vi "TDMS Read Channel Fields.vi"(4 "MN":string, 6 "SN":string, 7 "Group Name":string, 8 "error in (no error)":errorcluster, 9 "Channel":string, 10 "Custom Field Records to Search":string[](array[string]), 11 "tdms file ref":refnum<k34>) -> (0 "error out":errorcluster, 2 "Custom Fields":T1[](array[typedef]), 3 "tdms file ref":refnum<k34>)   [LabVIEW 2011]
uses:
  database/Fields/Field Record.ctl
  database/Fields/Field DataTypes.ctl
  database/Fields/Field NextItem.ctl
panel:
  out "x-y 2":u32
  out "x-y":u32
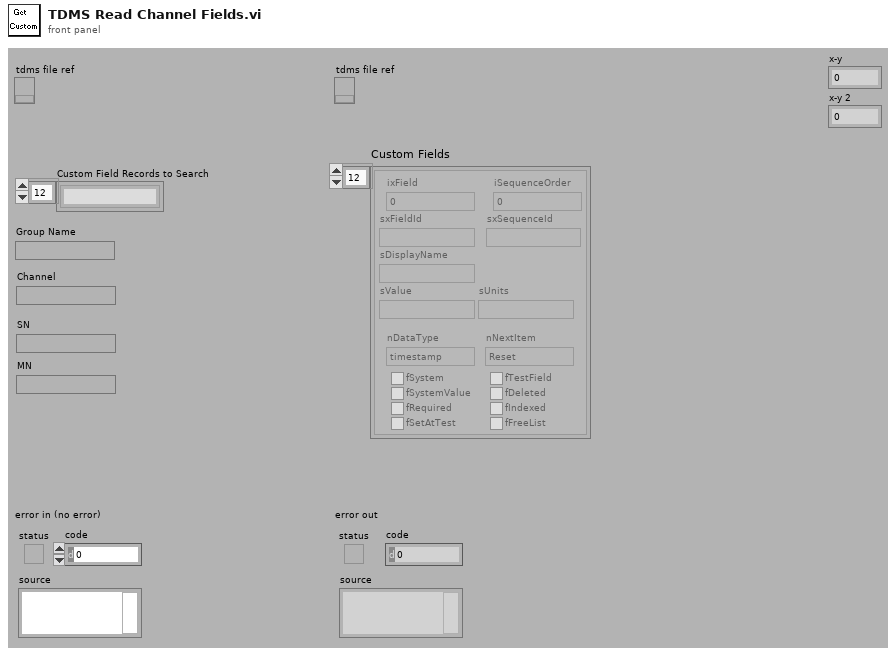
[diagram p1: front panel]
types:
  T1 = typedef "Field Record.ctl" = cluster{"ixField":i32, "iSequenceOrder":i32, "sxFieldId":string, "sxSequenceId":string, "sDisplayName":string, "sValue":string, "sUnits":string, "nDataType":T2, "nNextItem":T3, "fSystem":bool, "fSystemValue":bool, "fRequired":bool, "fSetAtTest":bool, "fTestField":bool, "fDeleted":bool, "fIndexed":bool, "fFreeList":bool}
  T2 = typedef "Field DataTypes.ctl" = enum32{"text", "numeric", "list", "timestamp", "boolean"}
  T3 = typedef "Field NextItem.ctl" = enum32{"Reset", "Retain", "Auto-Increment"}
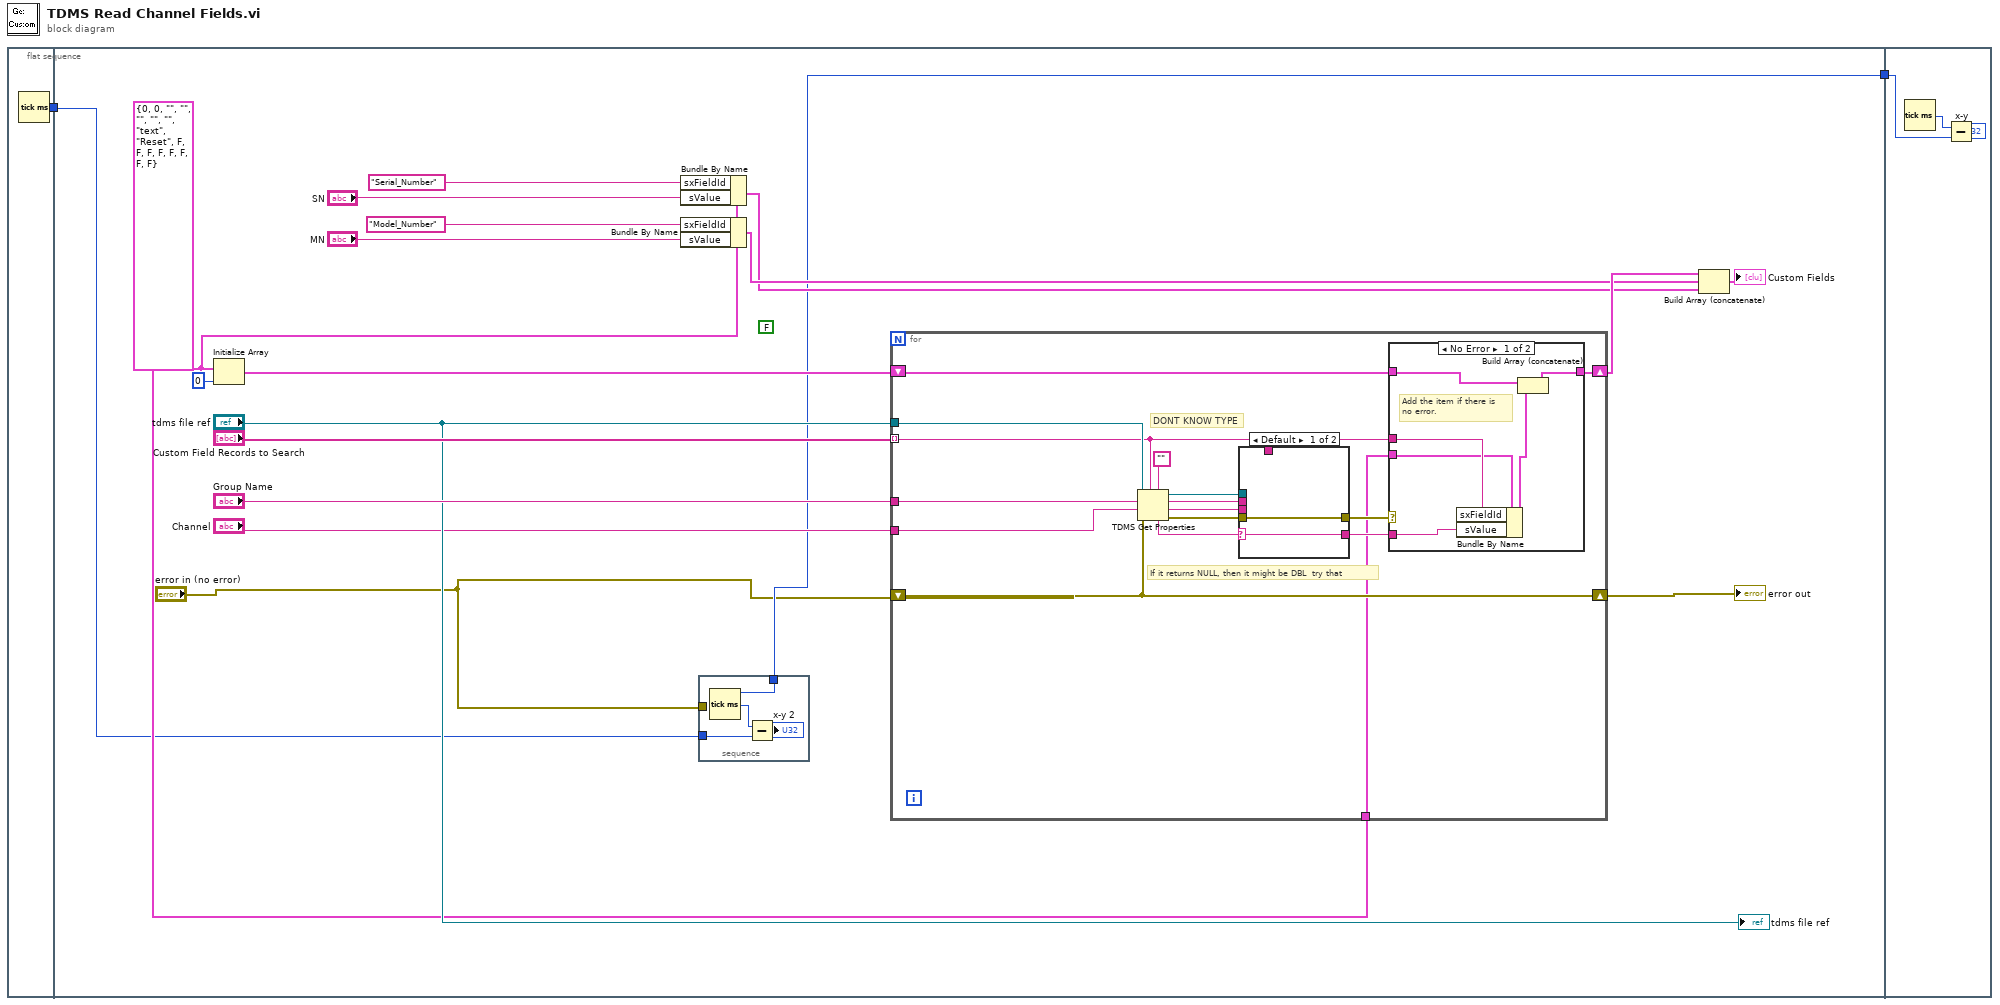
[diagram p0: block diagram]
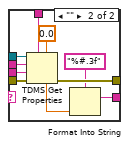
[diagram p2: hidden frame]
diagram:
  n1 = flat-sequence {
    tunnel: [w3] -> w1
    tunnel: [w6] -> w2
    tunnel: w1 -> [w5]
    tunnel: w2 -> [w62]
    frame #0 {
      n2 = Tick Count (ms)() -> (millisecond timer value=w3:u32)
    }
    frame #1 {
      (unwired) FALSE
      w15 = T1 {"ixField"=0, "iSequenceOrder"=0, "sxFieldId"="", "sxSequenceId"="", "sDisplayName"="", "sValue"="", "sUnits"="", "nDataType"=enum."text", "nNextItem"=enum."Reset", "fSystem"=FALSE, "fSystemValue"=FALSE, "fRequired"=FALSE, "fSetAtTest"=FALSE, "fTestField"=FALSE, "fDeleted"=FALSE, "fIndexed"=FALSE, "fFreeList"=FALSE} ("Field Record")
      n3 = Initialize Array(w15, 0 ("dimension size")) -> (w22:T1[])
      n4 = Bundle By Name(cluster=w15, "sxFieldId"="Serial_Number", "sValue"="SN") -> (w7:T1)
      n5 = Bundle By Name(cluster=w15, "sxFieldId"="Model_Number", "sValue"="MN") -> (w8:T1)
      n6 = stacked-sequence {
        tunnel: "error in (no error)" -> [_]
        tunnel: [w60] -> w6
        tunnel: w5 -> [w59]
        frame #0 {
          n7 = Tick Count (ms)() -> (millisecond timer value=w60:u32)
          n8 = Subtract(x=w60, y=w59) -> (x-y=→"x-y 2":u32)
        }
      }
      n9 = for {
        shift-right: [w36] -> w20
        shift-left: "error in (no error)" -> [w36]
        shift-right: [w37] -> w9
        shift-left: w22 -> [w38]
        tunnel: "tdms file ref" -> [w33]
        tunnel: "Custom Field Records to Search" -> [w30] mode=indexing
        tunnel: "Group Name" -> [w34]
        tunnel: w15 -> [w29]
        tunnel: "Channel" -> [w31]
        # "DONT KNOW TYPE"
        # "If it returns NULL, then it might be DBL  try that"
        n10 = TDMS Get Properties(5:"", 7:w30, 8:w36, 9:w31, 10:w34, 11:w33) -> (0:w27:errorcluster, 1:w23:string, 2:w24:string, 3:w26:refnum<k34>, 4:w25:string)  [unwired: 1 out]
        n11 = case shown="Default" w25 {
          selector: w25 -> [w39 _]
          tunnel: w27 -> [w40 w50]
          tunnel: w26 -> [_ w49]
          tunnel: w30 -> [_ w48]
          tunnel: [w40 w47] -> w32
          tunnel: [w39 w44] -> w35
          tunnel: w24 -> [_ w43]
          tunnel: w23 -> [_ w42]
          frame Default {
          }
          frame "" {
            n12 = TDMS Get Properties(5:0.0, 7:w48, 8:w50, 9:w42, 10:w43, 11:w49) -> (0:w47:errorcluster, 4:w46:dbl)  [unwired: 4 out]
            n13 = Format Into String(format string="%#.3f", w46) -> (resulting string=w44:string)  [unwired: 2 in, 1 out]
          }
        }
        n14 = case shown="No Error" w32 {
          tunnel: w38 -> [w56 w57]
          tunnel: [w55 w57] -> w37
          tunnel: w35 -> [w53 _]
          tunnel: w30 -> [w52 _]
          tunnel: w29 -> [w51 _]
          frame No Error {
            # "Add the item if there is\nno error."
            n15 = Bundle By Name(cluster=w51, "sxFieldId"=w52, "sValue"=w53) -> (w54:T1)
            n16 = Build Array (concatenate)(w56, w54) -> (w55:T1[])
          }
          frame Error {
          }
        }
      }
      "error out" <- w20
      n17 = Build Array (concatenate)(w9, w8, w7) -> (→"Custom Fields":T1[])
      "tdms file ref" <- "tdms file ref"
    }
    frame #2 {
      n18 = Tick Count (ms)() -> (millisecond timer value=w63:u32)
      n19 = Subtract(x=w63, y=w62) -> (x-y=→"x-y":u32)
    }
  }
